vi "Timer.vi"(8 "stop":bool) -> (3 "Elapsed time":dbl format="%#_3g")   [LabVIEW 2023]
panel:
  out "Zwro Time":dbl format="%#_3g"
  in  "Reset":bool
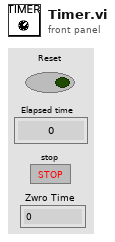
[diagram p1: front panel]
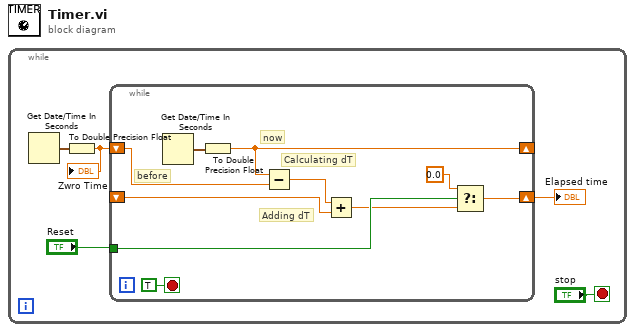
[diagram p0: block diagram]
diagram:
  n1 = while {
    stop <- "stop" stop-if-true
    n2 = Get Date/Time In Seconds() -> (seconds since 1Jan1904=w4:timestamp)
    n3 = To Double Precision Float(number=w4) -> (double precision float=w1:dbl)
    "Zwro Time" <- w1
    n4 = while {
      shift-right: [w10] -> _
      shift-left: w1 -> [w14]
      shift-right: [w8] -> w5
      shift-left: _ -> [w6]
      tunnel: "Reset" -> [w9]
      stop <- TRUE stop-if-true
      # "before"
      # "now"
      # "Adding dT"
      # "Calculating dT"
      n5 = Get Date/Time In Seconds() -> (seconds since 1Jan1904=w15:timestamp)
      n6 = To Double Precision Float(number=w15) -> (double precision float=w10:dbl)
      n7 = Subtract(x=w10, y=w14) -> (x-y=w13:dbl)
      n8 = Add(x=w13, y=w6) -> (x+y=w7:dbl)
      n9 = Select(t=0.0, s=w9, f=w7) -> (s? t:f=w8:dbl)
    }
    "Elapsed time" <- w5
  }
